vi "SweepRateConversion.vi"(1 "RAMP rate in":dbl, 2 "T/min to A/s (True)":bool) -> (0 "RAMP rate out":dbl)   [LabVIEW 2021]
doc: "converts Tesla/min to Amp/sec and vice versa :\n\nTrue = converts Tesla/min to Amp/sec\nFalse = converts Amp/sec to Tesla/min"
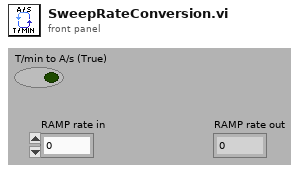
[diagram p1: front panel]
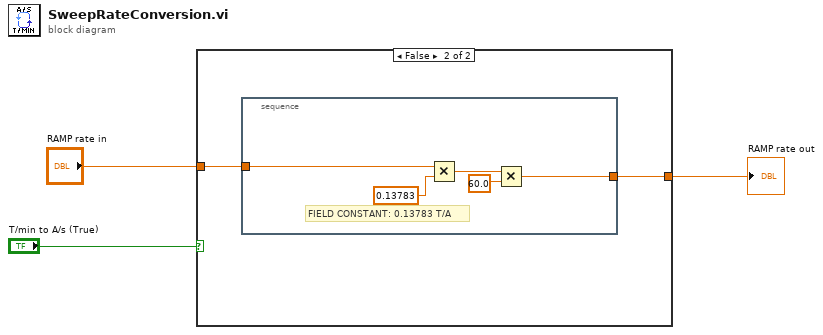
[diagram p0: block diagram]
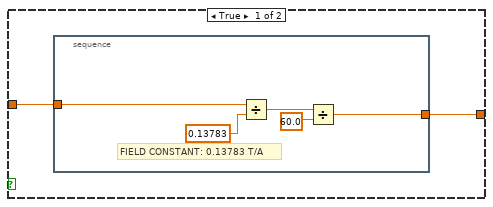
[diagram p2: hidden frame]
diagram:
  n1 = case shown="False" "T/min to A/s (True)" {
    tunnel: [w5 w12] -> w3
    tunnel: "RAMP rate in" -> [w4 w11]
    frame True {
      n2 = stacked-sequence {
        tunnel: [w7] -> w5
        tunnel: w4 -> [w6]
        frame #0 {
          # "FIELD CONSTANT: 0.13783 T/A"
          n3 = Divide(x=w6, y=0.13783) -> (x/y=w9:dbl)
          n4 = Divide(x=w9, y=60.0) -> (x/y=w7:dbl)
        }
      }
    }
    frame False {
      n5 = stacked-sequence {
        tunnel: [w14] -> w12
        tunnel: w11 -> [w13]
        frame #0 {
          # "FIELD CONSTANT: 0.13783 T/A"
          n6 = Multiply(x=w13, y=0.13783) -> (x*y=w16:dbl)
          n7 = Multiply(x=w16, y=60.0) -> (x*y=w14:dbl)
        }
      }
    }
  }
  "RAMP rate out" <- w3
